vi "Move_Files.vi"(7 "Run":string, 8 "PMTs":string[](array[string]), 9 "Channel":string[](array[string]), 10 "Folder Containing Bash Script":string="Wavedump_Bash_Script_Test_", 11 "Name of Folder to\nCopy PMT File to":string) -> ()   [LabVIEW 2018]
panel:
  out "File exists":bool
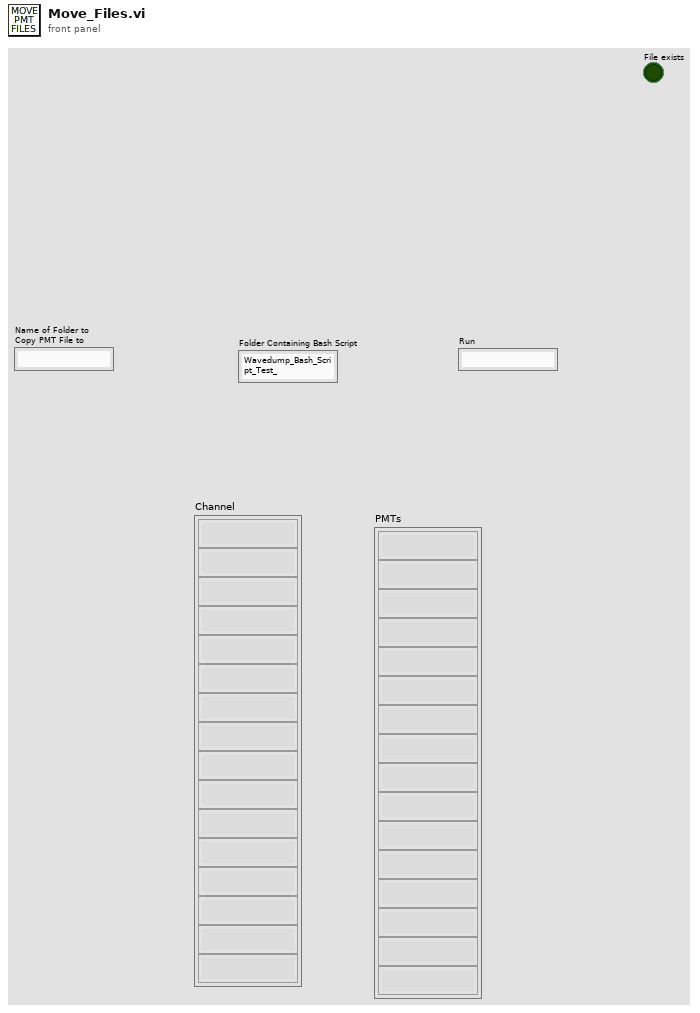
[diagram p1: front panel]
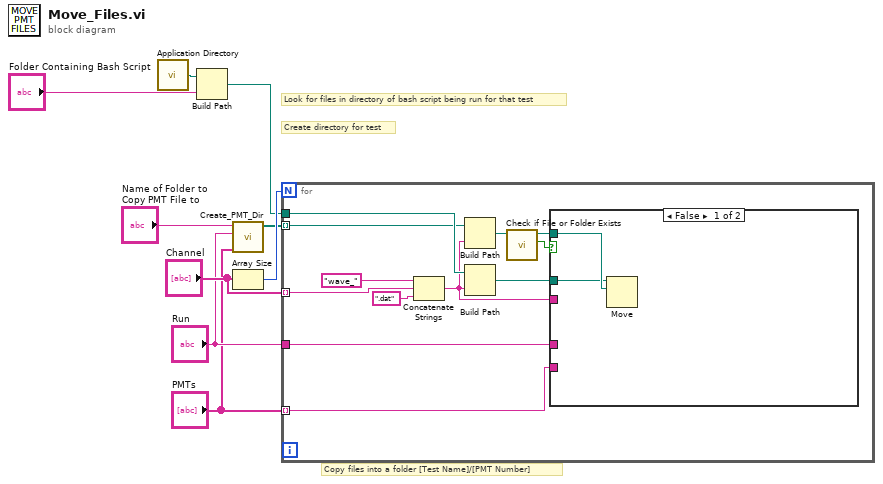
[diagram p0: block diagram]
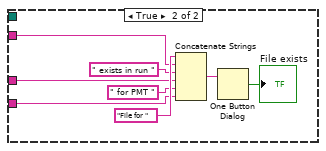
[diagram p2: hidden frame]
diagram:
  # "Create directory for test"
  # "Look for files in directory of bash script being run for that test"
  # "Copy files into a folder [Test Name]/[PMT Number]"
  n1 = call <vilib>:"Application Directory.vi"() -> ("Application Directory"=w9:path)
  n2 = Build Path(base path=w9, name or relative path="Folder Containing Bash Script") -> (appended path=w3:path)
  n3 = call "Create_PMT_Dir.vi"("Test"="Name of Folder to\nCopy PMT File to", "Run"="Run", "PMTs"="PMTs") -> ("Paths"=w5:path[])  [unwired: 7 in]
  n4 = Array Size(array="Channel") -> (size(s)=w6:i32)
  n5 = for {
    N: w6 -> [_]
    tunnel: w5 -> [w12] mode=indexing
    tunnel: w3 -> [w17]
    tunnel: "Channel" -> [w21] mode=indexing
    tunnel: "Run" -> [w16]
    tunnel: "PMTs" -> [w15] mode=indexing
    n6 = Concatenate Strings("wave_" ("string"), w21, ".dat" ("string")) -> (w10:string)
    n7 = Build Path(base path=w12, name or relative path=w10) -> (appended path=w11:path)
    n8 = Build Path(base path=w17, name or relative path=w10) -> (appended path=w14:path)
    n9 = call <vilib>:"Check if File or Folder Exists.vi"("path"=w11) -> ("file or folder exists?"=w20:bool, "dup path"=w13:path)  [unwired: 8 in, 1 out]
    n10 = case shown="False" w20 {
      tunnel: w13 -> [w23 _]
      tunnel: w14 -> [w22 _]
      tunnel: w10 -> [_ w29]
      tunnel: w16 -> [_ w27]
      tunnel: w15 -> [_ w25]
      frame False {
        n11 = Move(source path=w22, 10:w23) -> ()  [unwired: 3 in, 3 out]
      }
      frame True {
        n12 = Concatenate Strings("File for " ("string"), w29, " exists in run " ("string"), w27, " for PMT " ("string"), w25) -> (w24:string)
        n13 = One Button Dialog(message=w24) -> (true=→"File exists":bool)  [unwired: 1 in]
      }
    }
  }
